vi "MB cmd buffer.vi"(5 "MB cmd buffer":T4, 7 "Time":dbl format="%.2f", 8 "MB response in":dbl[](array[numeric]), 9 "MB ID-Address in":T1, 10 "ProCoDA Request in":T2 {"# registers" min=1}) -> (0 "wait":i32, 1 "output value":dbl, 2 "MB ID-Address out":T1, 3 "ProCoDA Request out":T2 {"# registers" min=1})   [LabVIEW 2019]
uses:
  MB cmd buffer.ctl
  ProCoDA MB Request.ctl
  Read Write.ctl
  MB ID-Address.ctl
panel:
  out "Last Updates":dbl[](array[numeric])
  out "MB responses out":dbl[][](array[numeric])
  out "New cmd out":bool[](array[boolean])
  out "Devices":T1[](array[typedef])
  out "ProCoDA Requests":T2[](array[typedef]) {"# registers" min=1}
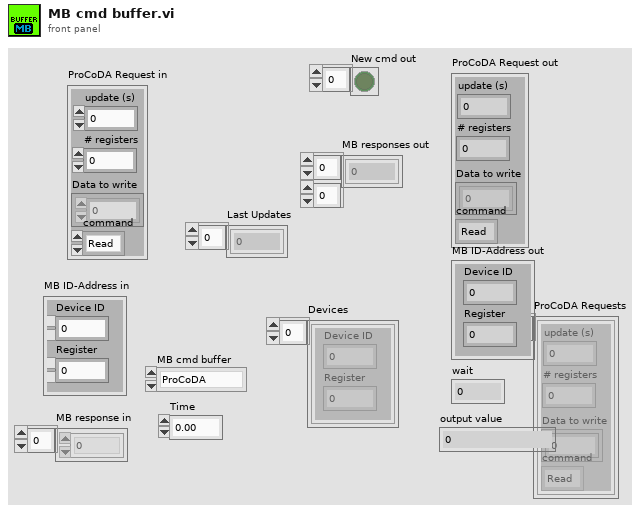
[diagram p1: front panel]
types:
  T1 = typedef "MB ID-Address.ctl" = cluster{"Device ID":u8, "Register":u16}
  T2 = typedef "ProCoDA MB Request.ctl" = cluster{"# registers":u8, "Data to write":u16[], "update (s)":dbl, "command":T3}
  T3 = typedef "Read Write.ctl" = enum16{"Read", "Write"}
  T4 = typedef "MB cmd buffer.ctl" = enum16{"ProCoDA", "MB", "MB Next Task", "ProCoDA read 1"}
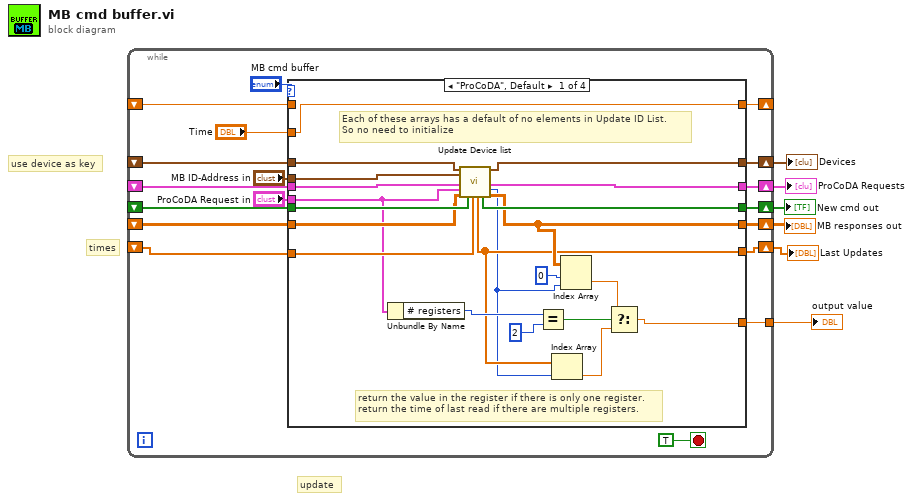
[diagram p0: block diagram]
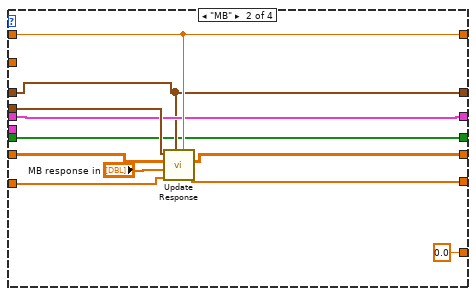
[diagram p2: hidden frame]
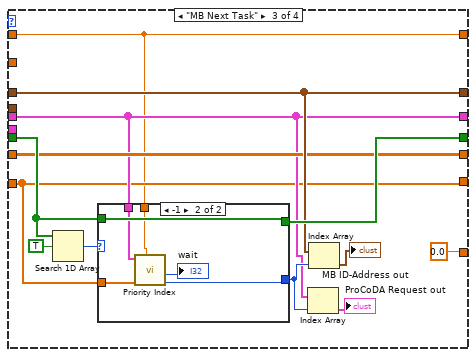
[diagram p3: hidden frame]
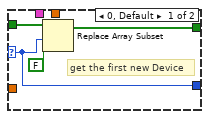
[diagram p4: hidden frame]
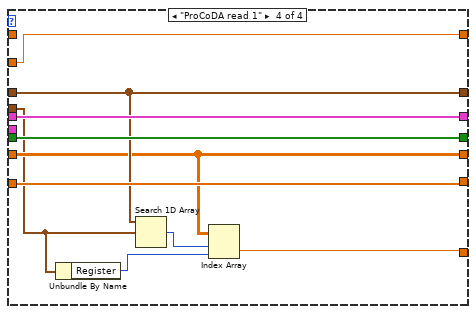
[diagram p5: hidden frame]
diagram:
  # "times"
  # "use device as key"
  # "update"
  n1 = while {
    shift-right: [w21] -> w5
    shift-left: _ -> [w22]
    shift-right: [w19] -> w6
    shift-left: _ -> [w20]
    shift-right: [w18] -> w4
    shift-left: _ -> [w17]
    shift-right: [w11] -> w2
    shift-left: _ -> [w16]
    shift-right: [w13] -> _
    shift-left: _ -> [w12]
    shift-right: [w10] -> w3
    shift-left: _ -> [w9]
    tunnel: [w8] -> w1
    stop <- TRUE stop-if-true
    n2 = case shown="\"ProCoDA\", Default" "MB cmd buffer" {
      tunnel: w22 -> [w43 w49 w60 w89]
      tunnel: [w42 w49 w60 w89] -> w21
      tunnel: w20 -> [w44 w48 w65 w86]
      tunnel: [w45 w48 w65 w86] -> w19
      tunnel: [w41 w47 w66 w88] -> w18
      tunnel: w17 -> [w40 w47 w67 w88]
      tunnel: w16 -> [w38 w55 w61 w85]
      tunnel: "ProCoDA Request in" -> [w32 _ _ _]
      tunnel: "MB ID-Address in" -> [w39 w56 _ w83]
      tunnel: [w27 w50 w58 w80] -> w13
      tunnel: w12 -> [_ w50 w58 _]
      tunnel: [w33 w54 w61 w85] -> w11
      tunnel: [w30 w52 w59 w87] -> w10
      tunnel: w9 -> [w37 w51 w59 w87]
      tunnel: [w28 0.0 ("Numeric") 0.0 ("Numeric") w81] -> w8
      tunnel: "Time" -> [w27 _ _ w80]
      frame "ProCoDA", Default {
        # "return the value in the register if there is only one register.\nreturn the time of last read if there are multiple registers."
        # "Each of these arrays has a default of no elements in Update ID List.\nSo no need to initialize"
        n3 = Unbundle By Name(w32) -> ("# registers"=w31:u8)
        n4 = call "Update Device list.vi"("Devices in"=w44, "MB ID-Address"=w39, "ProCoDA Requests in"=w43, "ProCoDA Request"=w32, "MB responses in"=w38, "New cmd in"=w40, "Last Updates in"=w37) -> ("Last Updates out"=w30:dbl[], "New cmd out"=w41:bool[], "Devices out"=w45:T1[], "ProCoDA Requests out"=w42:T2[], "index"=w25:i32, "MB responses out"=w33:dbl[][])  [unwired: 7 in]
        n5 = Equal?(x=w31, y=2) -> (x = y?=w35:bool)
        n6 = Index Array(array=w30, index=w25) -> (element=w29:dbl)
        n7 = Index Array(array=w33, index (row)=0 ("index"), index (col)=w25) -> (element=w34:dbl)
        n8 = Select(t=w34, s=w35, f=w29) -> (s? t:f=w28:dbl)
      }
      frame "MB" {
        n9 = call "Update Response.vi"("Time"=w50, "Devices in"=w48, "Last Updates in"=w51, "MB response in"="MB response in", "MB responses in"=w55, "MB ID-Address"=w56) -> ("Last Updates out"=w52:dbl[], "MB responses out"=w54:dbl[][])  [unwired: 4 in]
      }
      frame "MB Next Task" {
        n10 = Search 1D Array(1D array=w67, element=TRUE) -> (index of element=w68:i32)  [unwired: 1 in]
        n11 = case shown="-1" w68 {
          selector: w68 -> [w72 _]
          tunnel: [w72 w76] -> w63
          tunnel: w67 -> [w73 w79]
          tunnel: [w70 w79] -> w66
          tunnel: w60 -> [_ w78]
          tunnel: w59 -> [_ w77]
          tunnel: w58 -> [_ w75]
          frame 0, Default {
            # "get the first new Device"
            n12 = Replace Array Subset(array=w73, new element=FALSE ("new element/subarray"), index=w72) -> (w70:bool[])
          }
          frame -1 {
            n13 = call "Priority Index.vi"("Time"=w75, "Last Updates"=w77, "ProCoDA Requests"=w78) -> ("Priority Index"=w76:i32, "wait (ms)"=→"wait":i32)  [unwired: 7 in]
          }
        }
        n14 = Index Array(array=w60, index=w63) -> (element=→"ProCoDA Request out":T2)
        n15 = Index Array(array=w65, index=w63) -> (element=→"MB ID-Address out":T1)
      }
      frame "ProCoDA read 1" {
        n16 = Unbundle By Name(w83) -> ("Register"=w82:u16)
        n17 = Search 1D Array(1D array=w86, element=w83) -> (index of element=w84:i32)  [unwired: 1 in]
        n18 = Index Array(array=w85, index (row)=w84, index (col)=w82) -> (element=w81:dbl)
      }
    }
  }
  "ProCoDA Requests" <- w5
  "Devices" <- w6
  "New cmd out" <- w4
  "MB responses out" <- w2
  "Last Updates" <- w3
  "output value" <- w1
